vi "Global Simulated Arm Pot.vi"() -> ()   [LabVIEW 2017]
panel:
  in  "Simulated Arm Pot":dbl
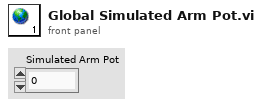
[diagram p1: front panel]
diagram:
